vi "Adaptive_not_icl.vi"() -> ()   [LabVIEW 2018]
uses:
  <vilib>/Analysis/_algsub.llb/Vector Norm.vi
  <vilib>/Analysis/_algsub.llb/Real Vector Norm.vi
  <vilib>/Analysis/baseanly.llb/Outer Product.vi
  <vilib>/Analysis/baseanly.llb/Real Outer Product.vi
  <vilib>/robotics/Kinematics/Create Lie Group Matrix.vi
  <vilib>/Analysis/baseanly.llb/Real Inverse Matrix.vi
  <vilib>/imath/engines/lvmath2/RunTimeEngine/NodeEndStatement/NIMS_NodeEndStatement_Output.vi
  <instcachedir>/0/NIMS_NodeEndStatement_Output_53EC0D466D134D7ABD903AC30B43404B.lvgen/NIMS_NodeEndStatement_Output_53EC0D466D134D7ABD903AC30B43404B_005.vi
  <instcachedir>/0/NIMS_NodeEndStatement_Output_53EC0D466D134D7ABD903AC30B43404B.lvgen/NIMS_NodeEndStatement_Output_53EC0D466D134D7ABD903AC30B43404B_000.vi
  <instcachedir>/0/NIMS_NodeEndStatement_Output_53EC0D466D134D7ABD903AC30B43404B.lvgen/NIMS_NodeEndStatement_Output_53EC0D466D134D7ABD903AC30B43404B_002.vi
  <vilib>/imath/engines/lvmath2/RunTimeEngine/ErrorHandling/NIMS_Finalize Error.vi
  <vilib>/Analysis/Matrix/Numeric/Conversions/Matrix To Array - RM.vi
  <vilib>/imath/engines/lvmath2/RunTimeEngine/IndexRead/NIMS M(S,S).vi
  <instcachedir>/0/NIMS M(S,S)_AC51E74150A542F7991B9634C66F3096.lvgen/NIMS M(S,S)_AC51E74150A542F7991B9634C66F3096_000.vi
  <vilib>/imath/engines/lvmath2/RunTimeEngine/BuiltInFunctions/abs/NIMS_abs(signed).vi
  <instcachedir>/0/NIMS_abs(signed)_C4FCB8E6058B49B797C7C8D53CA5F6EC.lvgen/NIMS_abs(signed)_C4FCB8E6058B49B797C7C8D53CA5F6EC_000.vi
  <vilib>/imathl/engines/lvmath/Functions/Error Handling/Create Error.vi
  <vilib>/imath/engines/lvmath2/RunTimeEngine/BuiltInFunctions/atan2/NIMS_atan2.vi
  <instcachedir>/0/NIMS_atan2_A91AA4A7D42247EDBE8F76DB99AF04A4.lvgen/NIMS_atan2_A91AA4A7D42247EDBE8F76DB99AF04A4_002.vi
  <vilib>/imath/engines/lvmath2/RunTimeEngine/ErrorHandling/NIMS_Create Error From Enums.vi
  <vilib>/imath/engines/lvmath2/RunTimeEngine/BuiltInFunctions/cos/NIMS_cos(C).vi
  <instcachedir>/0/NIMS_cos(C)_96B8A70E6B8E4D29AD8526A89C8CF3DF.lvgen/NIMS_cos(C)_96B8A70E6B8E4D29AD8526A89C8CF3DF_001.vi
  <instcachedir>/0/NIMS_atan2_A91AA4A7D42247EDBE8F76DB99AF04A4.lvgen/NIMS_atan2_A91AA4A7D42247EDBE8F76DB99AF04A4_001.vi
  <vilib>/imath/engines/lvmath2/RunTimeEngine/IndexRead/NIMS V(S).vi
  <instcachedir>/0/NIMS V(S)_0488751826AF41519A22953C041130DC.lvgen/NIMS V(S)_0488751826AF41519A22953C041130DC_000.vi
  <vilib>/imath/engines/lvmath2/RunTimeEngine/ArithmeticOperatorToken/NIMS_ArithmeticOperator_multmx(M,CV)-internal.vi
  <instcachedir>/0/NIMS_ArithmeticOperator_multmx(M,CV)-internal_5287250D8D1D4A3E9F77F5DF08D432E0.lvgen/NIMS_ArithmeticOperator_multmx(M,CV)-internal_5287250D8D1D4A3E9F77F5DF08D432E0_001.vi
  <vilib>/imath/engines/lvmath2/RunTimeEngine/ArithmeticOperatorToken/NIMS_ArithmeticOperator_multmx.vi
  <instcachedir>/0/NIMS_ArithmeticOperator_multmx_622CA76F9646436AB036D42A9A1CE0E6.lvgen/NIMS_ArithmeticOperator_multmx_622CA76F9646436AB036D42A9A1CE0E6_004.vi
  <vilib>/imath/engines/lvmath2/RunTimeEngine/ArithmeticOperatorToken/NIMS_ArithmeticOperator_minus.vi
  <instcachedir>/0/NIMS_ArithmeticOperator_minus_C4D0373119CC411691B2E50DF2E09F22.lvgen/NIMS_ArithmeticOperator_minus_C4D0373119CC411691B2E50DF2E09F22_002.vi
  <vilib>/imath/engines/lvmath2/RunTimeEngine/ArithmeticOperatorToken/NIMS_ArithmeticOperator_multmx(M,CV).vi
  <instcachedir>/0/NIMS_ArithmeticOperator_multmx(M,CV)_2F1CD6A2FE4F4213A4AD1C901C2750F5.lvgen/NIMS_ArithmeticOperator_multmx(M,CV)_2F1CD6A2FE4F4213A4AD1C901C2750F5_000.vi
  <vilib>/imath/engines/lvmath2/RunTimeEngine/BuiltInFunctions/inv/NIMS_inv(GM).vi
  <instcachedir>/0/NIMS_inv(GM)_A6DF8FE880224208AACFE4CF9F659502.lvgen/NIMS_inv(GM)_A6DF8FE880224208AACFE4CF9F659502_001.vi
  <vilib>/imath/engines/lvmath2/RunTimeEngine/ErrorHandling/NIMS_Error From Error Code.vi
  <instcachedir>/0/NIMS V(S)_0488751826AF41519A22953C041130DC.lvgen/NIMS V(S)_0488751826AF41519A22953C041130DC_003.vi
  <vilib>/imath/engines/lvmath2/RunTimeEngine/BuiltInFunctions/sin/NIMS_sin(C).vi
  <instcachedir>/0/NIMS_sin(C)_7FE83C8DCD97403BBE687635FA1F837E.lvgen/NIMS_sin(C)_7FE83C8DCD97403BBE687635FA1F837E_001.vi
  <vilib>/imath/engines/lvmath2/RunTimeEngine/IndexRead/NIMS M(S).vi
  <instcachedir>/0/NIMS M(S)_B826C018497E4940AE96BD27B540B6FB.lvgen/NIMS M(S)_B826C018497E4940AE96BD27B540B6FB_000.vi
  <vilib>/imath/engines/lvmath2/RunTimeEngine/RowToken/NIMS_RowToken_M_M.vi
  <instcachedir>/0/NIMS_RowToken_M_M_9381229BAB584C0281F245468A1A9A6C.lvgen/NIMS_RowToken_M_M_9381229BAB584C0281F245468A1A9A6C_003.vi
  <vilib>/imath/engines/lvmath2/RunTimeEngine/ArithmeticOperatorToken/NIMS_ArithmeticOperator_plus.vi
  <instcachedir>/0/NIMS_ArithmeticOperator_plus_DE670E32103C4C10ADF2A97367172B30.lvgen/NIMS_ArithmeticOperator_plus_DE670E32103C4C10ADF2A97367172B30_003.vi
  <instcachedir>/0/NIMS_ArithmeticOperator_multmx_622CA76F9646436AB036D42A9A1CE0E6.lvgen/NIMS_ArithmeticOperator_multmx_622CA76F9646436AB036D42A9A1CE0E6_007.vi
  <instcachedir>/0/NIMS_ArithmeticOperator_plus_DE670E32103C4C10ADF2A97367172B30.lvgen/NIMS_ArithmeticOperator_plus_DE670E32103C4C10ADF2A97367172B30_010.vi
  <instcachedir>/0/NIMS_ArithmeticOperator_multmx_622CA76F9646436AB036D42A9A1CE0E6.lvgen/NIMS_ArithmeticOperator_multmx_622CA76F9646436AB036D42A9A1CE0E6_003.vi
  <vilib>/imath/engines/lvmath2/RunTimeEngine/ArithmeticOperatorToken/NIMS_ArithmeticOperator_multmx-internal.vi
  <instcachedir>/0/NIMS_ArithmeticOperator_multmx-internal_16A6E1DA326644AB974D30232E729C42.lvgen/NIMS_ArithmeticOperator_multmx-internal_16A6E1DA326644AB974D30232E729C42_001.vi
  <instcachedir>/0/NIMS_ArithmeticOperator_multmx(M,CV)_2F1CD6A2FE4F4213A4AD1C901C2750F5.lvgen/NIMS_ArithmeticOperator_multmx(M,CV)_2F1CD6A2FE4F4213A4AD1C901C2750F5_003.vi
  <instcachedir>/0/NIMS_ArithmeticOperator_plus_DE670E32103C4C10ADF2A97367172B30.lvgen/NIMS_ArithmeticOperator_plus_DE670E32103C4C10ADF2A97367172B30_002.vi
  <vilib>/imath/engines/lvmath2/RunTimeEngine/MatrixToken/NIMS_MatrixToken_M_SorCV.vi
  <instcachedir>/0/NIMS_MatrixToken_M_SorCV_91F8B6182BA1450B95B3875CCE45F523.lvgen/NIMS_MatrixToken_M_SorCV_91F8B6182BA1450B95B3875CCE45F523_000.vi
  <instcachedir>/0/NIMS_ArithmeticOperator_multmx(M,CV)_2F1CD6A2FE4F4213A4AD1C901C2750F5.lvgen/NIMS_ArithmeticOperator_multmx(M,CV)_2F1CD6A2FE4F4213A4AD1C901C2750F5_002.vi
  <vilib>/imath/engines/lvmath2/RunTimeEngine/NodeEndStatement/NIMS_NodeEndStatement_Get Vector.vi
  <instcachedir>/0/NIMS_NodeEndStatement_Get Vector_329D0992E87F49F089135171B7FC9327.lvgen/NIMS_NodeEndStatement_Get Vector_329D0992E87F49F089135171B7FC9327_003.vi
  <vilib>/imath/engines/lvmath/Functions/Error Handling/MergeErrorsWrapper.vi
  <instcachedir>/0/NIMS_NodeEndStatement_Output_53EC0D466D134D7ABD903AC30B43404B.lvgen/NIMS_NodeEndStatement_Output_53EC0D466D134D7ABD903AC30B43404B_003.vi
  <instcachedir>/0/NIMS_ArithmeticOperator_multmx(M,CV)-internal_5287250D8D1D4A3E9F77F5DF08D432E0.lvgen/NIMS_ArithmeticOperator_multmx(M,CV)-internal_5287250D8D1D4A3E9F77F5DF08D432E0_004.vi
  <instcachedir>/0/NIMS_ArithmeticOperator_minus_C4D0373119CC411691B2E50DF2E09F22.lvgen/NIMS_ArithmeticOperator_minus_C4D0373119CC411691B2E50DF2E09F22_008.vi
  <instcachedir>/0/NIMS_ArithmeticOperator_minus_C4D0373119CC411691B2E50DF2E09F22.lvgen/NIMS_ArithmeticOperator_minus_C4D0373119CC411691B2E50DF2E09F22_009.vi
  <instcachedir>/0/NIMS_ArithmeticOperator_multmx_622CA76F9646436AB036D42A9A1CE0E6.lvgen/NIMS_ArithmeticOperator_multmx_622CA76F9646436AB036D42A9A1CE0E6_008.vi
  <instcachedir>/0/NIMS M(S)_B826C018497E4940AE96BD27B540B6FB.lvgen/NIMS M(S)_B826C018497E4940AE96BD27B540B6FB_004.vi
  <vilib>/imath/engines/lvmath2/RunTimeEngine/Managers/WorkSpace/UID Generator.vi
  <vilib>/imath/engines/lvmath2/RunTimeEngine/RunTimeType/NIMS_RunTimeType_From StrictType (excl LVString).vi
  <instcachedir>/0/NIMS_RunTimeType_From StrictType (excl LVString)_E7E34A65C99947108168652BAD14964D.lvgen/NIMS_RunTimeType_From StrictType (excl LVString)_E7E34A65C99947108168652BAD14964D_000.vi
  <vilib>/imath/engines/lvmath2/RunTimeEngine/LocalVariableDefStatement/MC_LocalVariableDefStatement_Display.vi
  <vilib>/imath/engines/lvmath2/RunTimeEngine/Managers/SymbolTable/Clear UID.vi
  <vilib>/Analysis/Matrix/Numeric/Multiply/Multiply.vi
  <vilib>/Analysis/Matrix/Numeric/Multiply/Multiply - RM,R.vi
  <vilib>/Analysis/Matrix/Numeric/Multiply/Multiply - R,RM.vi
  <vilib>/Analysis/Matrix/Numeric/Add/Add.vi
  <vilib>/Analysis/Matrix/Numeric/Add/Add - RM,RM.vi
  <instcachedir>/0/NIMS_NodeEndStatement_Output_53EC0D466D134D7ABD903AC30B43404B.lvgen/NIMS_NodeEndStatement_Output_53EC0D466D134D7ABD903AC30B43404B_001.vi
  <instcachedir>/0/NIMS_NodeEndStatement_Output_53EC0D466D134D7ABD903AC30B43404B.lvgen/NIMS_NodeEndStatement_Output_53EC0D466D134D7ABD903AC30B43404B_008.vi
  <vilib>/imath/engines/lvmath2/RunTimeEngine/IndexRead/NIMS M($,S).vi
  <instcachedir>/0/NIMS M($,S)_3E5749BBB62E49528D4765A77F1F6D98.lvgen/NIMS M($,S)_3E5749BBB62E49528D4765A77F1F6D98_000.vi
  <vilib>/imath/engines/lvmath2/RunTimeEngine/RowToken/NIMS_RowToken_SorRV_CV.vi
  <instcachedir>/0/NIMS_RowToken_SorRV_CV_E9A223509C5746E8B9F22970C86A52C1.lvgen/NIMS_RowToken_SorRV_CV_E9A223509C5746E8B9F22970C86A52C1_000.vi
  <vilib>/imath/engines/lvmath2/RunTimeEngine/IndexRead/NIMS V(R2).vi
  <instcachedir>/0/NIMS V(R2)_C76619605A0E4E9F8B2FA9389712AC47.lvgen/NIMS V(R2)_C76619605A0E4E9F8B2FA9389712AC47_000.vi
  <vilib>/imath/engines/lvmath2/RunTimeEngine/BuiltInFunctions/mean/NIMS_RS=mean(RV,I32).vi
  <vilib>/Analysis/NI_AALBase.lvlib
  <vilib>/gmath/NI_Gmath.lvlib
  <vilib>/Analysis/Matrix/NI_Matrix.lvlib
  <vilib>/robotics/Kinematics/NI_Kinematics.lvlib
  <vilib>/imath/engines/lvmath2/RunTimeEngine/Managers/SymbolTable/NIMS_WorkSpace.lvlib
panel:
  out "avg_er3":dbl
  out "avg_er2":dbl
  out "avg_er1":dbl
  out "eR (Yaw)":cluster{"E1_now":dbl[], "t_now":dbl[]}(graph)
  out "eR (Pitch)":cluster{"E1_now":dbl[], "t_now":dbl[]}(graph)
  out "eR (Roll)":cluster{"E1_now":dbl[], "t_now":dbl[]}(graph)
  out "Yaw":cluster{"E1_now":dbl[], "t_now":dbl[]}(graph)
  out "Pitch":cluster{"E1_now":dbl[], "t_now":dbl[]}(graph)
  out "Roll":cluster{"E1_now":dbl[], "t_now":dbl[]}(graph)
  in  "MOI(kg*m^2)":dbl[][](array[numeric])
  in  "COG(m)":dbl[](array[numeric])
  in  "Mass (kg)":dbl
  in  "Simulation Time(sec)":dbl
  # "Physical Parameters"
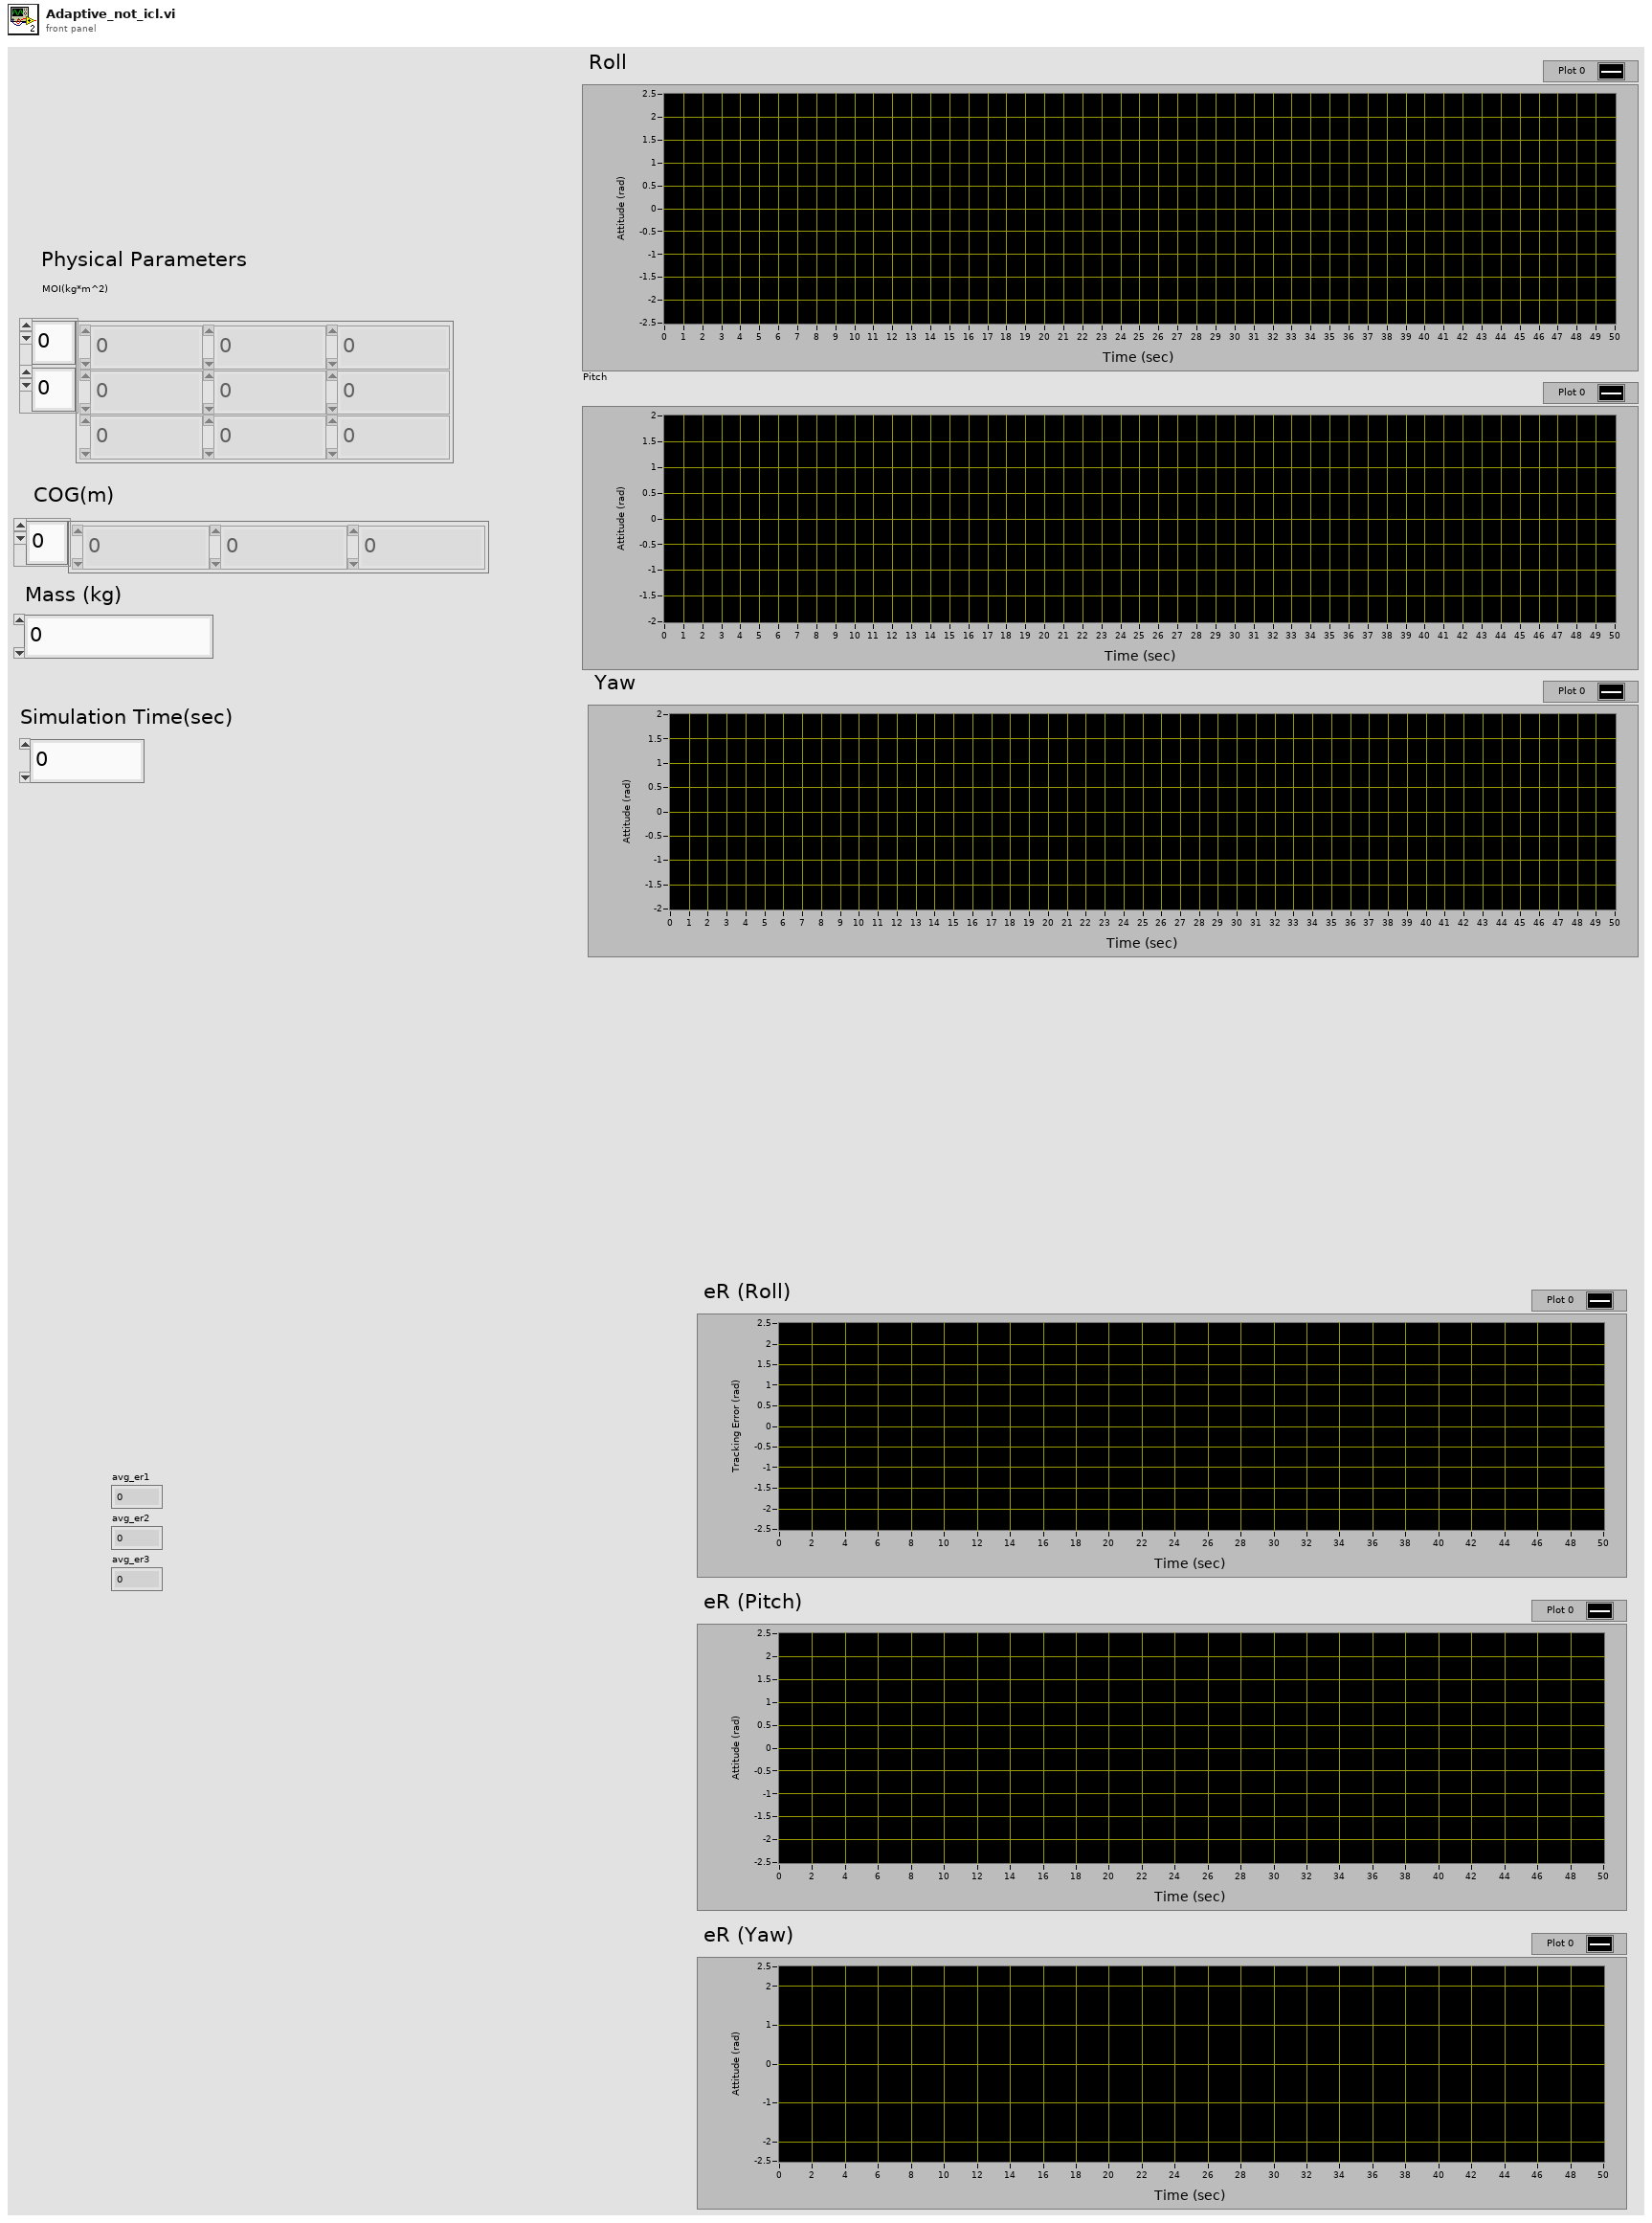
[diagram p1: front panel]
types:
  T1 = cluster{"Er1":dbl[], "Er2":dbl[], "Er3":dbl[], "t":dbl[]}
  T2 = cluster{"E1":cdb[], "E2":dbl[], "E3":dbl[], "t":dbl[]}
  T3 = typedef "NI_Matrix.lvlib/RealMatrix.ctl" = dbl[][]
  T4 = typedef "NI_Kinematics.lvlib/Quaternion.ctl" = dbl[]
  T5 = cluster{"E1_now":cdb[], "E2_now":cdb[], "E3_now":dbl[], "t_now":dbl[]}
  T6 = cluster{"Er1":dbl[], "Er2":dbl[], "Er3":dbl[], "t_now":dbl[]}
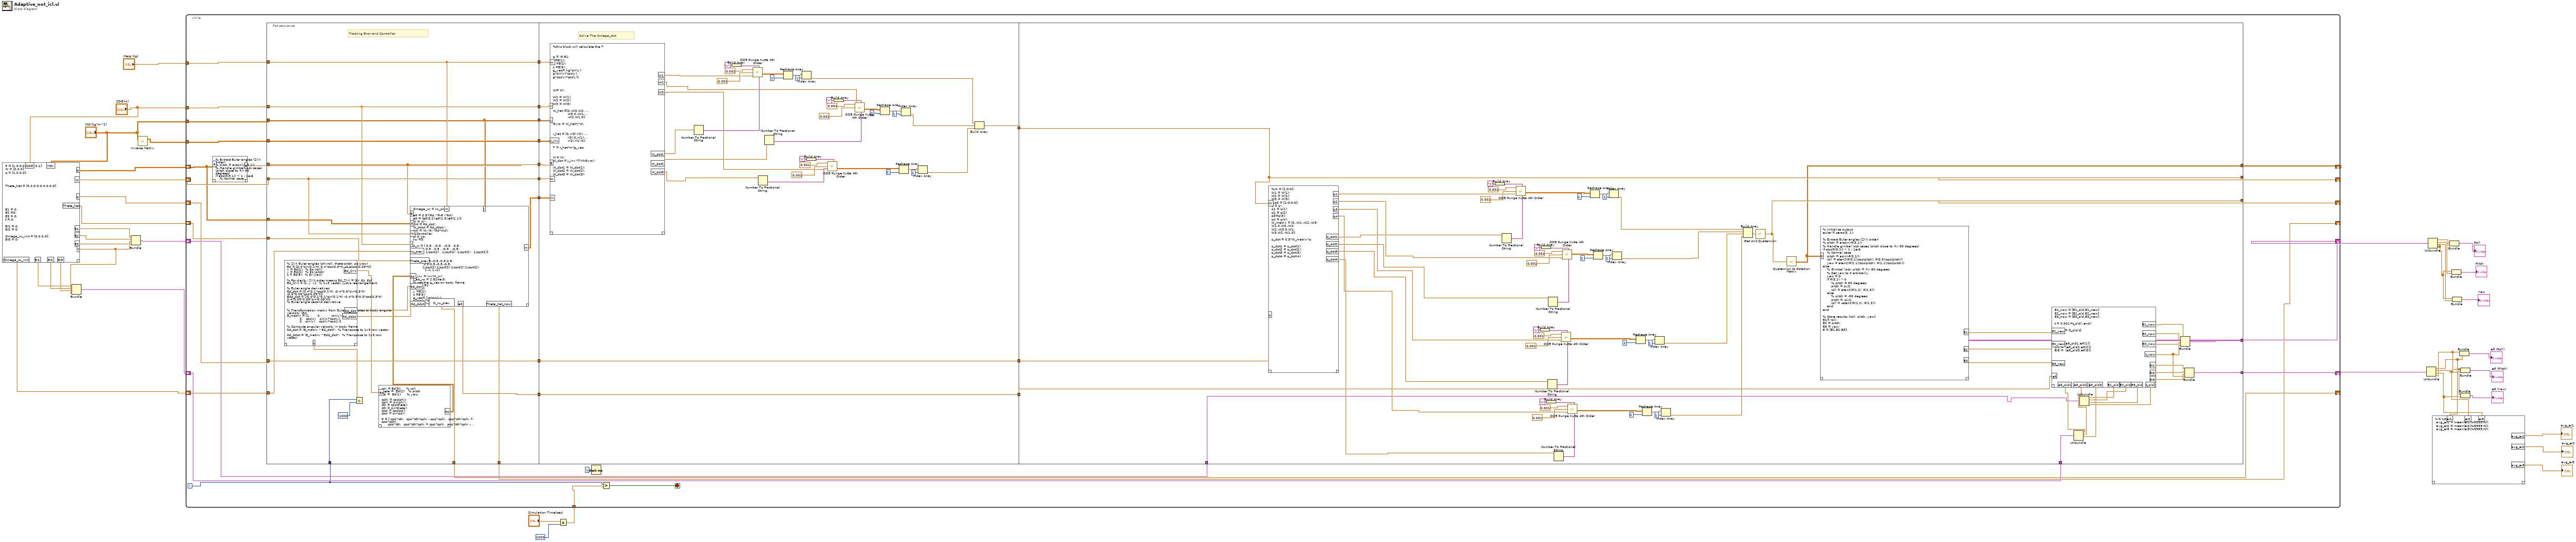
[diagram p0: block diagram]
diagram:
  n1 = mathscript code="R = [1,0,0;0,1,0;0,0,1];\nW = [0,0,0];\nq = [1,0,0,0];\n\n\n\nTheta_hat = [0,0,0,0,0,0,0,0,0];\n\n\n\n\n\n\nE1 = 0;\nE2 =0;\nE3 = 0;\nt = 0;\n\nEr1 = 0;\nEr2 = 0;\n\nOmega_rw_init = [0,0,0,0];\nEr3 = 0;"("MOI"="MOI(kg*m^2)", "COG"="COG(m)") -> ("R"=w35:dbl[][], "W"=w34:dbl[], "q"=w33:dbl[], "E1"=w32:cdb[], "E2"=w31:dbl[], "E3"=w30:dbl[], "t"=w12:dbl[], "Er1"=w21:dbl[], "Er2"=w20:dbl[], "Er3"=w19:dbl[], "Omega_rw_init"=w4:dbl[], "Theta_hat"=w1:dbl[])  [unwired: 1 in, 1 out]
  n2 = Bundle("Er1"=w21, "Er2"=w20, "Er3"=w19, "t"=w12) -> (w18:T1)  [unwired: 1 in]
  n3 = Bundle("E1"=w32, "E2"=w31, "E3"=w30, "t"=w12) -> (w29:T2)  [unwired: 1 in]
  n4 = call-poly <vilib>:"Inverse Matrix.vi"("Input Matrix"="MOI(kg*m^2)") -> ("Inverse Matrix"=w36:T3)  [unwired: 1 in, 1 out]
  n5 = Multiply(x="Simulation Time(sec)", y=1000) -> (x*y=w38:dbl)
  n6 = while {
    tunnel: w38 -> [w62]
    tunnel: "Mass (kg)" -> [w71]
    tunnel: "COG(m)" -> [w72]
    tunnel: w36 -> [w74]
    tunnel: "MOI(kg*m^2)" -> [w73]
    shift-right: [w65] -> _
    shift-left: w35 -> [w51]
    shift-right: [w64] -> _
    shift-left: w34 -> [w70]
    shift-right: [w66] -> _
    shift-left: w33 -> [w67]
    shift-right: [w60] -> w28
    shift-left: w29 -> [w61]
    shift-right: [w45] -> w17
    shift-left: w18 -> [w46]
    shift-right: [w42] -> _
    shift-left: w4 -> [w44]
    shift-right: [w41] -> _
    shift-left: w1 -> [w43]
    i -> [w50]
    stop <- w63 stop-if-true
    n7 = mathscript code="% Extract Euler angles (ZYX order)\n% pitch = arcsin(-R(3,1))\n% Handle gimbal lock cases (pitch close to +/- 90 degrees)\nif abs(R(3,1)) < 1 - 1e-6\n    % Normal case\n    pitch = asin(-R(3,1));\n    roll = atan2(R(3,2)/cos(pitch), R(3,3)/cos(pitch));\n    yaw = atan2(R(2,1)/cos(pitch), R(1,1)/cos(pitch));\nelse\n    % Gimbal lock: pitch = +/- 90 degrees\n    % Set yaw to 0 arbitrarily\n    yaw = 0;\n    if R(3,1) < 0\n        % pitch = 90 degrees\n        pitch = pi/2;\n        roll = atan2(R(1,2), R(1,3));\n    else\n        % pitch = -90 degrees\n        pitch = -pi/2;\n        roll = -atan2(R(1,2), R(1,3));\n    end\nend\n\n% Store results: [roll, pitch, yaw]\nE1= roll;\nE2 = pitch;\nE3 = yaw;\nE = [E1,E2,E3];"("R"=w51) -> ("E"=w69:cdb[])  [unwired: 1 in, 1 out]
    n8 = flat-sequence {
      tunnel: w67 -> [w371]
      tunnel: w70 -> [w369]
      tunnel: w71 -> [w363]
      tunnel: w72 -> [w365]
      tunnel: w73 -> [w362]
      tunnel: w74 -> [w372]
      tunnel: w69 -> [w364]
      tunnel: [w364] -> w58
      tunnel: [w372] -> w57
      tunnel: [w362] -> w56
      tunnel: [w365] -> w55
      tunnel: [w363] -> w54
      tunnel: [w369] -> w53
      tunnel: [w371] -> w52
      tunnel: w51 -> [w370]
      tunnel: w50 -> [w368]
      tunnel: [w361] -> w49
      tunnel: [w356] -> w47
      tunnel: [w355] -> w42
      tunnel: w44 -> [w354]
      tunnel: w43 -> [w353]
      tunnel: [w352] -> w41
      tunnel: [w1985] -> w68
      tunnel: [w1984] -> w59
      tunnel: w58 -> [w2027]
      tunnel: w57 -> [w2026]
      tunnel: w56 -> [w2025]
      tunnel: w55 -> [w2024]
      tunnel: w54 -> [w2023]
      tunnel: w53 -> [w2022]
      tunnel: w52 -> [w1985]
      tunnel: w49 -> [w1983]
      tunnel: [w1982] -> w48
      tunnel: w47 -> [w1982]
      tunnel: w68 -> [w2470]
      tunnel: [w2469] -> w66
      tunnel: [w2467] -> w65
      tunnel: [w2468] -> w64
      tunnel: w61 -> [w2460]
      tunnel: [w2456] -> w60
      tunnel: w59 -> [w2468]
      tunnel: w48 -> [w2454]
      tunnel: w46 -> [w2449]
      tunnel: [w2450] -> w45
      frame #0 {
        # "Tracking Error and Controller"
        n9 = Divide(x=w368, y=1000) -> (x/y=w360:dbl)
        n10 = mathscript code="% ZYX Euler angles (phi-roll, theta-pitch, psi-yaw)\nEd = [0.4*sin(0.1*t); 0.4*cos(0.3*t); -0.4*sin(0.09*t)];  \nx = Ed(1);  % £p (roll)\ny = Ed(2);  % £c (pitch)\nz = Ed(3);  % £r (yaw)\n\n% For clarity: ZYX order means Ed_ZYX = [£r, £c, £p]\nEd_ZYX = [z, y, x];  % 1x3 vector, just a rearrangement\n\n% Euler angle derivatives\nEd_dot = [0.4*0.1*cos(0.1*t); -0.4*0.3*sin(0.3*t); -0.4*0.09*cos(0.09*t)];\nEdd_dot = [-0.4*0.1*0.1*sin(0.1*t); -0.4*0.3*0.3*cos(0.3*t); 0.4*0.09*0.09*sin(0.09*t)];\n% Euler angle second derivative\n\n\n% Transformation matrix from Euler angle rates to body angular velocity (£s)\nE_matrix = [1,       0,          -sin(y);\n            0,   cos(x),   sin(x)*cos(y);\n            0,  -sin(x),   cos(x)*cos(y)];\n\n% Compute angular velocity in body frame\nRd_dot = (E_matrix * Ed_dot)';  % Transpose to 1x3 row vector\n\nRd_ddot = (E_matrix * Edd_dot)';  % Transpose to 1x3 row vector"("t"=w360) -> ("Ed_ZYX"=w359:dbl[], "Rd_dot"=w366:dbl[], "Rd_ddot"=w357:dbl[])  [unwired: 1 in, 1 out]
        n11 = mathscript code="phi = Ed(3);     % roll\ntheta =  Ed(2);   % pitch\npsi =  Ed(1);     % yaw\n\ncphi = cos(phi);\nsphi = sin(phi);\ncth = cos(theta);\nsth = sin(theta);\ncpsi = cos(psi);\nspsi = sin(psi);\n\nR = [ cpsi*cth,  cpsi*sth*sphi - spsi*cphi,  cpsi*sth*cphi + spsi*sphi;\n      spsi*cth,  spsi*sth*sphi + cpsi*cphi,  spsi*sth*cphi - cpsi*sphi;\n      -sth,      cth*sphi,                  cth*cphi ];\nRd = R;"("Ed"=w359) -> ("Rd"=w358:dbl[][])  [unwired: 1 in, 1 out]
        n12 = mathscript code="Omega_rw = rw_prev';\n\neR = 0.5*(Rd.'*R-R.'*Rd);\neR = [eR(3,2);eR(1,3);eR(2,1)];\nW = W';\nWd = Rd_dot';\nW_ddot = Rd_ddot.';\neW = W- (R.'*Rd*Wd);\n%Controller\nkr = 10;\nkw =3;\n\nA_w = [ 0.5 , -0.5 , -0.5 , 0.5;\n            0.5 , 0.5 , -0.5 , -0.5;\n            1/sqrt(2) , 1/sqrt(2) ,1/sqrt(2) , 1/sqrt(2)];\n\n\nH_w = [0.5,-0.5,-0.5,0.5;\n          0.5,0.5,-0.5,-0.5;\n         1/sqrt(2),1/sqrt(2),1/sqrt(2),1/sqrt(2);\n           1,-1,1,-1];\n\nH_inv = inv(H_w);\nJ_ab_rw = 2.824e-3;\n% get the g_vec on body frame\ng = -9.81;\nx=E(1);\ny =E(2);\nz =E(3);\ng_vec= [-g*sin(y);\ng*sin(x)*cos(y);\ng*cos(x)*cos(y)];\n\n\n\nW1 = W(1);\nW2 = W(2);\nW3 = W(3);\n\nW_hat =[0,-W3,W2;...\n              W3,0,-W1;...\n              -W2,W1,0];\n\nr_hat = [0,-r(3),r(2); ...\n              r(3),0,-r(1);...\n              -r(2),r(1),0];\n\n%maintain_term\n%J*(W_hat*R.'*Rd*Wd)\n\n%Regression matrix\ng_1 =g_vec(1);\ng_2 = g_vec(2);\ng_3 = g_vec(3);\n\n\nY_cog = [0,-m*g_3,m*g_2 ;\n              m*g_3,0,-m*g_1;\n               -m*g_2,m*g_1,0];\n\nW_bar =W_hat*R'*Rd*Wd-R'*Rd*W_ddot;\nY_J = [-W_bar(1),W_bar(1)*W_bar(3),-W_bar(1)*W_bar(2);\n         -W_bar(2)*W_bar(3),-W_bar(2),W_bar(1)*W_bar(2);\nW_bar(2)*W_bar(3),-W_bar(1)*W_bar(3),-W_bar(3);\n-W_bar(2)-W_bar(1)*W_bar(3), -W_bar(1)-W_bar(2)*W_bar(3),-W_bar(2)*W_bar(2)+W_bar(1)*W_bar(1);\n-W_bar(3)-W_bar(1)*W_bar(2),-W_bar(1)*W_bar(1)+W_bar(3)*W_bar(3),-W_bar(1)-W_bar(2)*W_bar(3);\n(W_bar(2)*W_bar(2))-(W_bar(3)*W_bar(3)),-W_bar(3)-W_bar(1)*W_bar(2),-W_bar(2)-W_bar(1)*W_bar(3)];\nY_J = Y_J';\n\nY_sys =[Y_J, Y_cog];\n\ngamma = 0.01;\n\n% Adaptive ctrol law\nTheta_hat_dot = gamma* Y_sys'*(eW+eR);\n\nTheta_hat_prev = Theta_prev';\nTheta_hat = Theta_hat_prev+Theta_hat_dot*0.001;\n\nTheta_hat_now = Theta_hat';\n\n\n\n\n\n\n%M_G = -kr*eR-kw*eW+W_hat*J*W-r_hat*m*g_vec-J*(W_hat*R.'*Rd*Wd-R.'*Rd*W_ddot);\nM_G = -kr*eR-kw*eW+Y_sys*Theta_hat+W_hat*A_w*J_ab_rw*Omega_rw;\n%M = M';\nM_RW_com = [M_G;0];\nOmega_dot = -(H_inv/J_ab_rw)*M_RW_com;\nOmega_rw_now =Omega_rw+ Omega_dot*0.001;\nM = A_w*J_ab_rw*Omega_dot+W_hat*A_w*J_ab_rw*Omega_rw_now;\nM =M';\n%M = [0.0,0.0,0.0];\neR = [eR(1),eR(2),eR(3)];\neW = [eW(1),eW(2),eW(3)];\n\nO_rw_prev = Omega_rw_now';"("R"=w370, "W"=w369, "Rd"=w358, "Rd_dot"=w366, "r"=w365, "E"=w364, "m"=w363, "J"=w362, "Rd_ddot"=w357, "rw_prev"=w354, "Theta_prev"=w353) -> ("M"=w361:cdb[][], "eR"=w356:dbl[], "O_rw_prev"=w355:dbl[], "Theta_hat_now"=w352:dbl[])  [unwired: 1 in, 1 out]
      }
      frame #1 {
        # "Solve The Omega_dot"
        n13 = mathscript code="%this block will calculate the T\n\n\ng = -9.81;\nx=E(1);\ny =E(2);\nz =E(3);\ng_vec= [-g*sin(y);\ng*sin(x)*cos(y);\ng*cos(x)*cos(y)];\n\n\n\nW= W';\n\nW1 = W(1);\nW2 = W(2);\nW3 = W(3);\n\nW_hat =[0,-W3,W2; ...\n              W3,0,-W1;...\n              -W2,W1,0];\n\nGyro = W_hat*J*W;\n\n\nr_hat = [0,-r(3),r(2); ...\n              r(3),0,-r(1);...\n              -r(2),r(1),0];\n\nT = r_hat*m*g_vec;\n\n\nM = M';\nW_dot = J_inv*(T-M-Gyro);\n\nW_dot1 = W_dot(1);\nW_dot2 = W_dot(2);\nW_dot3 = W_dot(3);"("E"=w2027, "J"=w2025, "J_inv"=w2026, "r"=w2024, "m"=w2023, "W"=w2022, "M"=w1983) -> ("W_dot1"=w1986:dbl[], "W_dot2"=w1987:dbl[], "W_dot3"=w1988:dbl[], "W1"=w1991:dbl[], "W2"=w1990:dbl[], "W3"=w1989:dbl[])  [unwired: 1 in, 1 out]
        n14 = Number To Fractional String(number=w1986) -> (F-format string=w2017:string[])  [unwired: 3 in]
        n15 = Build Array("x") -> (w2020:string[])
        n16 = call <vilib>:"ODE Runge Kutta 4th Order.vi"("time end"=0.001, "h (step rate)"=0.001, "X0"=w1991, "X (name of variables)"=w2020, "F(X,t) (right sides of the ODE\nas functions of X and t)"=w2017) -> ("X Values (solution)"=w2013:dbl[][])  [unwired: 2 in, 3 out]
        n17 = Number To Fractional String(number=w1988) -> (F-format string=w1999:string[])  [unwired: 3 in]
        n18 = Number To Fractional String(number=w1987) -> (F-format string=w2008:string[])  [unwired: 3 in]
        n19 = Reshape Array(w2013, 2 ("dimension size")) -> (w2015:dbl[])
        n20 = Index Array(array=w2015, index=1) -> (element=w1994:dbl)
        n21 = Build Array("x") -> (w2002:string[])
        n22 = call <vilib>:"ODE Runge Kutta 4th Order.vi"("time end"=0.001, "h (step rate)"=0.001, "X0"=w1989, "X (name of variables)"=w2002, "F(X,t) (right sides of the ODE\nas functions of X and t)"=w1999) -> ("X Values (solution)"=w1995:dbl[][])  [unwired: 2 in, 3 out]
        n23 = Build Array("x") -> (w2011:string[])
        n24 = call <vilib>:"ODE Runge Kutta 4th Order.vi"("time end"=0.001, "h (step rate)"=0.001, "X0"=w1990, "X (name of variables)"=w2011, "F(X,t) (right sides of the ODE\nas functions of X and t)"=w2008) -> ("X Values (solution)"=w2004:dbl[][])  [unwired: 2 in, 3 out]
        n25 = Reshape Array(w2004, 2 ("dimension size")) -> (w2006:dbl[])
        n26 = Reshape Array(w1995, 2 ("dimension size")) -> (w1997:dbl[])
        n27 = Index Array(array=w2006, index=1) -> (element=w1993:dbl)
        n28 = Index Array(array=w1997, index=1) -> (element=w1992:dbl)
        n29 = Build Array(w1994, w1993, w1992) -> (w1984:dbl[])
      }
      frame #2 {
        n30 = mathscript code="%W = [1;0;0];\nW1 = W(1);\nW2 = W(2);\nW3 = W(3);\n%q0 = [1;0;0;0];\nq = q';\nq1 = q(1);\nq2 = q(2)\nq3=q(3);\nq4 = q(4);\nW_matrix = [0,-W1,-W2,-W3;\nW1,0,W3,-W2;\nW2,-W3,0,W1;\nW3,W2,-W1,0];\n\nq_dot = 0.5*W_matrix*q;\n\nq_dot1 = q_dot(1);\nq_dot2 = q_dot(2);\nq_dot3 = q_dot(3);\nq_dot4 = q_dot(4);"("q"=w2470, "W"=w2468) -> ("q_dot1"=w2509:dbl[], "q_dot2"=w2498:dbl[], "q_dot3"=w2487:dbl[], "q_dot4"=w2476:dbl[], "q1"=w2510:dbl[], "q2"=w2499:dbl[], "q3"=w2488:dbl[], "q4"=w2477:dbl[])  [unwired: 1 in, 1 out]
        n31 = Build Array("x") -> (w2518:string[])
        n32 = Number To Fractional String(number=w2509) -> (F-format string=w2515:string[])  [unwired: 3 in]
        n33 = call <vilib>:"ODE Runge Kutta 4th Order.vi"("time end"=0.001, "h (step rate)"=0.001, "X0"=w2510, "X (name of variables)"=w2518, "F(X,t) (right sides of the ODE\nas functions of X and t)"=w2515) -> ("X Values (solution)"=w2511:dbl[][])  [unwired: 2 in, 3 out]
        n34 = Build Array("x") -> (w2496:string[])
        n35 = Build Array("x") -> (w2507:string[])
        n36 = Build Array("x") -> (w2485:string[])
        n37 = Number To Fractional String(number=w2487) -> (F-format string=w2493:string[])  [unwired: 3 in]
        n38 = Number To Fractional String(number=w2498) -> (F-format string=w2504:string[])  [unwired: 3 in]
        n39 = Number To Fractional String(number=w2476) -> (F-format string=w2482:string[])  [unwired: 3 in]
        n40 = call <vilib>:"ODE Runge Kutta 4th Order.vi"("time end"=0.001, "h (step rate)"=0.001, "X0"=w2488, "X (name of variables)"=w2496, "F(X,t) (right sides of the ODE\nas functions of X and t)"=w2493) -> ("X Values (solution)"=w2489:dbl[][])  [unwired: 2 in, 3 out]
        n41 = call <vilib>:"ODE Runge Kutta 4th Order.vi"("time end"=0.001, "h (step rate)"=0.001, "X0"=w2499, "X (name of variables)"=w2507, "F(X,t) (right sides of the ODE\nas functions of X and t)"=w2504) -> ("X Values (solution)"=w2500:dbl[][])  [unwired: 2 in, 3 out]
        n42 = call <vilib>:"ODE Runge Kutta 4th Order.vi"("time end"=0.001, "h (step rate)"=0.001, "X0"=w2477, "X (name of variables)"=w2485, "F(X,t) (right sides of the ODE\nas functions of X and t)"=w2482) -> ("X Values (solution)"=w2478:dbl[][])  [unwired: 2 in, 3 out]
        n43 = Reshape Array(w2511, 2 ("dimension size")) -> (w2513:dbl[])
        n44 = Reshape Array(w2500, 2 ("dimension size")) -> (w2502:dbl[])
        n45 = Index Array(array=w2513, index=1) -> (element=w2475:dbl)
        n46 = Index Array(array=w2502, index=1) -> (element=w2474:dbl)
        n47 = Reshape Array(w2489, 2 ("dimension size")) -> (w2491:dbl[])
        n48 = Reshape Array(w2478, 2 ("dimension size")) -> (w2480:dbl[])
        n49 = Index Array(array=w2491, index=1) -> (element=w2473:dbl)
        n50 = Index Array(array=w2480, index=1) -> (element=w2472:dbl)
        n51 = Build Array(w2475, w2474, w2473, w2472) -> (w2471:dbl[])
        n52 = call <vilib>:"Get Unit Quaternion.vi"("quaternion"=w2471) -> ("unit quaternion"=w2469:T4)
        n53 = call <vilib>:"Quaternion to Rotation Matrix.vi"("quaternion"=w2469) -> ("rotation matrix"=w2467:T3)
        n54 = mathscript code="% Initialize output\neuler = zeros(3, 1);\n\n% Extract Euler angles (ZYX order)\n% pitch = arcsin(-R(3,1))\n% Handle gimbal lock cases (pitch close to +/- 90 degrees)\nif abs(R(3,1)) < 1 - 1e-6\n    % Normal case\n    pitch = asin(-R(3,1));\n    roll = atan2(R(3,2)/cos(pitch), R(3,3)/cos(pitch));\n    yaw = atan2(R(2,1)/cos(pitch), R(1,1)/cos(pitch));\nelse\n    % Gimbal lock: pitch = +/- 90 degrees\n    % Set yaw to 0 arbitrarily\n    yaw = 0;\n    if R(3,1) < 0\n        % pitch = 90 degrees\n        pitch = pi/2;\n        roll = atan2(R(1,2), R(1,3));\n    else\n        % pitch = -90 degrees\n        pitch = -pi/2;\n        roll = -atan2(R(1,2), R(1,3));\n    end\nend\n\n% Store results: [roll, pitch, yaw]\nE1= roll;\nE2 = pitch;\nE3 = yaw;\nE = [E1,E2,E3];"("R"=w2467) -> ("E1"=w2466:dbl, "E2"=w2465:cdb, "E3"=w2464:dbl)  [unwired: 1 in, 1 out]
        n55 = Unbundle(w2449) -> ("Er1"=w2448:dbl[], "Er2"=w2447:dbl[], "Er3"=w2446:dbl[])  [unwired: 1 out]
        n56 = Unbundle(w2460) -> ("E1_now"=w2463:cdb[], "E2_now"=w2462:cdb[], "E3_now"=w2461:dbl[], "t_now"=w2455:dbl[])
        n57 = mathscript code="E1_now = [E1_old,E1_new];\nE2_now = [E2_old,E2_new];\nE3_now = [E3_old,E3_new];\n\nt = 0.001+t_old(:,end);\n\nt_now = [t_old,t];\n\n\n\nEr1 = [eR_old1,eR(1)];\nEr2 =  [eR_old2,eR(2)];\nEr3 =  [eR_old3,eR(3)];"("E1_new"=w2466, "E2_new"=w2465, "E3_new"=w2464, "E1_old"=w2463, "E2_old"=w2462, "E3_old"=w2461, "t_old"=w2455, "eR"=w2454, "eR_old1"=w2448, "eR_old2"=w2447, "eR_old3"=w2446) -> ("E1_now"=w2459:cdb[], "E2_now"=w2458:cdb[], "E3_now"=w2457:dbl[], "t_now"=w2445:dbl[], "Er1"=w2453:dbl[], "Er2"=w2452:dbl[], "Er3"=w2451:dbl[])  [unwired: 1 in, 1 out]
        n58 = Bundle("E1_now"=w2459, "E2_now"=w2458, "E3_now"=w2457, "t_now"=w2445) -> (w2456:T5)  [unwired: 1 in]
        n59 = Bundle("Er1"=w2453, "Er2"=w2452, "Er3"=w2451, "t_now"=w2445) -> (w2450:T6)  [unwired: 1 in]
      }
    }
    n60 = Wait (ms)(milliseconds to wait=u32 1) -> ()  [unwired: 1 out]
    n61 = Greater?(x=w50, y=w62) -> (0:w63:bool)
  }
  n62 = Unbundle(w17) -> ("Er1"=w10:dbl[], "Er2"=w9:dbl[], "Er3"=w8:dbl[], "t_now"=w11:dbl[])
  n63 = Unbundle(w28) -> ("E1_now"=w27:cdb[], "E2_now"=w26:cdb[], "E3_now"=w13:dbl[], "t_now"=w25:dbl[])
  n64 = mathscript code="N = 10000;\n avg_er1 = mean(er1(N-9999:N));\n avg_er2 = mean(er2(N-9999:N));\n avg_er3 = mean(er3(N-9999:N));"("er1"=w10, "er2"=w9, "er3"=w8) -> ("avg_er1"=→"avg_er1":dbl, "avg_er2"=→"avg_er2":dbl, "avg_er3"=→"avg_er3":dbl)  [unwired: 1 in, 1 out]
  n65 = Bundle("t_now"=w25, "E1_now"=w27) -> (→"Roll":cluster{"t_now":dbl[], "E1_now":cdb[]})  [unwired: 1 in]
  n66 = Bundle("t_now"=w25, "E2_now"=w26) -> (→"Pitch":cluster{"t_now":dbl[], "E2_now":cdb[]})  [unwired: 1 in]
  n67 = Bundle("t_now"=w25, "E3_now"=w13) -> (→"Yaw":cluster{"t_now":dbl[], "E3_now":dbl[]})  [unwired: 1 in]
  n68 = Bundle("t_now"=w11, "Er1"=w10) -> (→"eR (Roll)":cluster{"t_now":dbl[], "Er1":dbl[]})  [unwired: 1 in]
  n69 = Bundle("t_now"=w11, "Er2"=w9) -> (→"eR (Pitch)":cluster{"t_now":dbl[], "Er2":dbl[]})  [unwired: 1 in]
  n70 = Bundle("t_now"=w11, "Er3"=w8) -> (→"eR (Yaw)":cluster{"t_now":dbl[], "Er3":dbl[]})  [unwired: 1 in]
